vi "GenNewTraj.vi"(8 "Stoopid Overlap %":dbl min=0.0, 10 "Parameters":T2={"Sample Period (s)"=0.0, "Limits"={"Velocity (fps)"=6.0, "Accel (fps^2)"=15.0, "Jerk (fps^3)"=150.0, "StoopidFast (fps)"=6.0}, "Conditions"={"vInitial (fps)"=0.0, "vFinal (fps)"=0.0}, "Overrides"=[]} {"Overrides"."Angular Multiplier 2" step=5.0; "Overrides"."Angular Multiplier" step=5.0; "Limits"."StoopidFast (fps)" min=0.0; "Limits"."Jerk (fps^3)" min=0.0 step=1.0; "Limits"."Accel (fps^2)" min=0.0; "Limits"."Velocity (fps)" min=0.0}, 11 "Points in":cluster{"x":dbl, "y":dbl, "th":dbl}[](array[cluster])) -> (0 "Time (s)":dbl, 1 "Valid":bool, 2 "Trajectory Data":T3(array[cluster]), 3 "Updated Waypoints":cluster{"x":dbl, "y":dbl, "th":dbl}[](array[cluster]), 4 "Distance (ft)":dbl)   [LabVIEW 2019]
uses:
  Types/Limits.ctl
  5b132355-d611-49ac-9db4-4ea5228ca0e8.vi
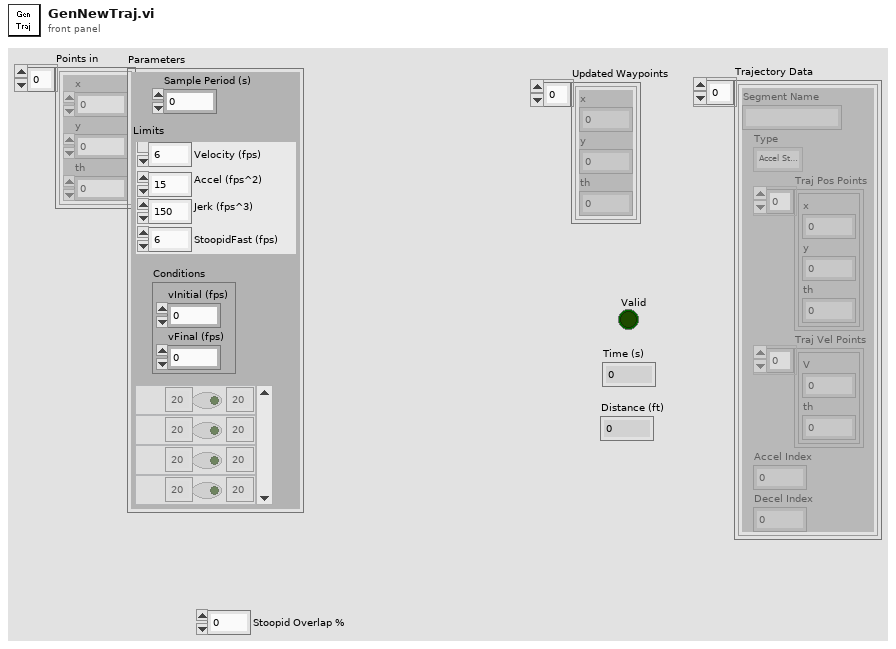
[diagram p1: front panel]
types:
  T1 = typedef "Limits.ctl" = cluster{"Velocity (fps)":dbl, "Accel (fps^2)":dbl, "Jerk (fps^3)":dbl, "StoopidFast (fps)":dbl}
  T2 = cluster{"Sample Period (s)":dbl, "Limits":T1, "Conditions":cluster{"vInitial (fps)":dbl, "vFinal (fps)":dbl}, "Overrides":cluster{"Count":string, "Angular Multiplier":dbl, "1":bool, "Angular Multiplier 2":dbl}[]}
  T3 = cluster{"Segment Name":string, "Type":enum16{"Accel Straight", "Const Straight", "Blend", "Circle"}, "Traj Pos Points":cluster{"x":dbl, "y":dbl, "th":dbl}[], "Traj Vel Points":cluster{"V":dbl, "th":dbl}[], "Accel Index":i32, "Decel Index":i32}[]
  T4 = cluster{"vInitial (fps)":dbl, "vFinal (fps)":dbl}
  T5 = cluster{"Count":string, "Angular Multiplier":dbl, "1":bool, "Angular Multiplier 2":dbl}[]
  T6 = cluster{"Points in":cluster{"x":dbl, "y":dbl, "th":dbl}[], "Sample Period (s)":dbl, "Limits":T1, "Conditions":cluster{"vInitial (fps)":dbl, "vFinal (fps)":dbl}, "Overrides":cluster{"Count":string, "Angular Multiplier":dbl, "1":bool, "Angular Multiplier 2":dbl}[]}
  T7 = cluster{"Trajectory Data":cluster{"Segment Name":string, "Type":enum16{"Accel Straight", "Const Straight", "Blend", "Circle"}, "Traj Pos Points":cluster{"x":dbl, "y":dbl, "th":dbl}[], "Traj Vel Points":cluster{"V":dbl, "th":dbl}[], "Accel Index":i32, "Decel Index":i32}[], "Time (s)":dbl, "Valid":bool, "Updated Waypoints":cluster{"x":dbl, "y":dbl, "th":dbl}[], "Distance (ft)":dbl}
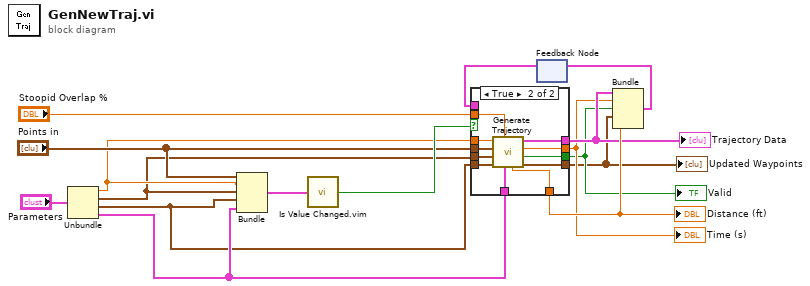
[diagram p0: block diagram]
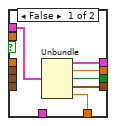
[diagram p2: hidden frame]
diagram:
  n1 = Unbundle("Parameters") -> ("Sample Period (s)"=w3:dbl, "Limits"=w2:T1, "Conditions"=w1:T4, "Overrides"=w5:T5)
  n2 = Bundle("Points in"="Points in", "Sample Period (s)"=w3, "Limits"=w2, "Conditions"=w1, "Overrides"=w5) -> (w7:T6)  [unwired: 1 in]
  n3 = call "Is Value Changed.vim"("value"=w7) -> ("changed or first call?"=w6:bool)
  n4 = feedback #1() -> (w15:T7)  [unwired: 1 in]
  n5 = case shown="True" w6 {
    tunnel: [w19 w33] -> w11
    tunnel: [w20 w32] -> w12
    tunnel: [w17 w31] -> w16
    tunnel: w1 -> [_ w30]
    tunnel: w2 -> [_ w29]
    tunnel: w5 -> [_ w28]
    tunnel: "Points in" -> [_ w27]
    tunnel: [w18 w26] -> w10
    tunnel: [w21 w25] -> w13
    tunnel: w3 -> [_ w24]
    tunnel: w15 -> [w22 _]
    tunnel: "Stoopid Overlap %" -> [_ w23]
    frame False {
      n6 = Unbundle(w22) -> ("Trajectory Data"=w21:T3, "Time (s)"=w20:dbl, "Valid"=w19:bool, "Updated Waypoints"=w18:cluster{"x":dbl, "y":dbl, "th":dbl}[], "Distance (ft)"=w17:dbl)
    }
    frame True {
      n7 = call "Generate Trajectory.vi"("Overrides 2"=w28, "Stoopid Overlap %"=w23, "Conditions"=w30, "Limits"=w29, "WayPoints"=w27, "Sample Period (s)"=w24) -> ("Updated Waypoints"=w26:cluster{"x":dbl, "y":dbl, "th":dbl}[], "Valid"=w33:bool, "Time (s)"=w32:dbl, "Trajectory Data"=w25:T3, "Distance (ft)"=w31:dbl)  [unwired: 1 in]
    }
  }
  "Distance (ft)" <- w16
  "Trajectory Data" <- w13
  "Time (s)" <- w12
  "Valid" <- w11
  "Updated Waypoints" <- w10
  n8 = Bundle("Trajectory Data"=w13, "Time (s)"=w12, "Valid"=w11, "Updated Waypoints"=w10, "Distance (ft)"=w16) -> (w14:T7)  [unwired: 1 in]
  n9 = feedback-in #1(w14) -> ()
